vi "ADXL345 I2C Open.vi"(8 "error in (no error)":errorcluster, 9 "Range":T3 items=["+/- 2 g", "+/- 4 g", "+/- 8 g", "+/- 16 g"], 11 "DIO Module (Slot 4)":T2=enum."Digital Module 2") -> (0 "error out":errorcluster, 3 "I2CDevRef":T1 {"Device Address" format="%.0x"})   [LabVIEW 2011]
uses:
  <vilib>/Rock Robotics/SystemInterfaces/Typedef/FPGA_TypedefDigitalModule.ctl
  ADXL345 I2C Range.ctl
  <vilib>/Rock Robotics/WPI/I2C/WPI_I2CDevRef.ctl
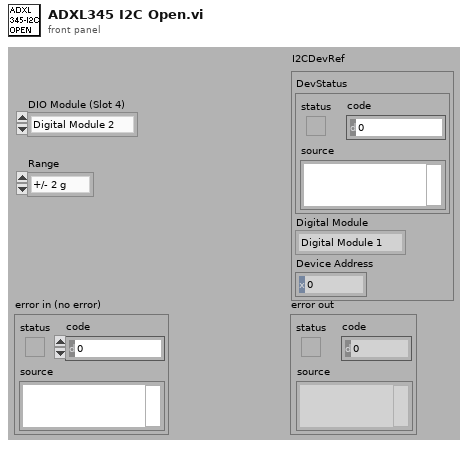
[diagram p1: front panel]
types:
  T1 = typedef "WPI_I2CDevRef.ctl" = cluster{"DevStatus":errorcluster, "Digital Module":T2, "Device Address":u8}
  T2 = typedef "FPGA_TypedefDigitalModule.ctl" = enum16{"Digital Module 1", "Digital Module 2"}
  T3 = typedef "ADXL345 I2C Range.ctl" = u8
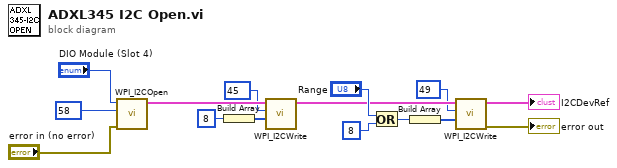
[diagram p0: block diagram]
diagram:
  n1 = call <vilib>:"WPI_I2COpen.vi"("error in (no error)"="error in (no error)", "Device Address"=u8 58 ("Data To Send"), "Digital Module (Module 1)"="DIO Module (Slot 4)") -> ("I2CDevRef"=w8:T1)  [unwired: 8 out]
  n2 = Build Array(u8 8 ("Data To Send")) -> (w5:u8[])
  n3 = call <vilib>:"WPI_I2CWrite.vi"("I2CDataToSend"=w5, "I2CRegister"=u8 45 ("Data To Send"), "I2CDevRef"=w8) -> ("I2CDevRef"=w11:T1)  [unwired: 2 in, 6 out]
  n4 = Or(x="Range", y=u8 8 ("Data To Send")) -> (x .or. y?=w4:T3)
  n5 = Build Array(w4) -> (w3:T3[])
  n6 = call <vilib>:"WPI_I2CWrite.vi"("I2CDataToSend"=w3, "I2CRegister"=u8 49 ("Data To Send"), "I2CDevRef"=w11) -> ("error out"=→"error out":errorcluster, "I2CDevRef"=→"I2CDevRef":T1)  [unwired: 2 in, 5 out]
